vi "run_script-as_admin.vi"(8 "error in (no error)":errorcluster, 11 "script_command":string) -> (0 "error out":errorcluster)   [LabVIEW 2015, in "lv-bin-windows.lvlib" / "v1.lvlib"]
uses:
  v1.lvlib
  <userlib>/antonio-alexander/lv-bin/lv-bin/public/api/v1/v1.lvlib
  lv-bin-windows.lvlib
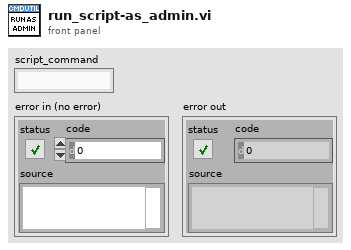
[diagram p1: front panel]
types:
  T1 = enum16{"open", "replace", "create", "open or create", "replace or create", "replace or create with confirmation"}
  T2 = typedef "lv-bin.lvlib/v1.lvlib/temp_dir_config.ctl" = cluster{"root_folder":path, "prefix":string}
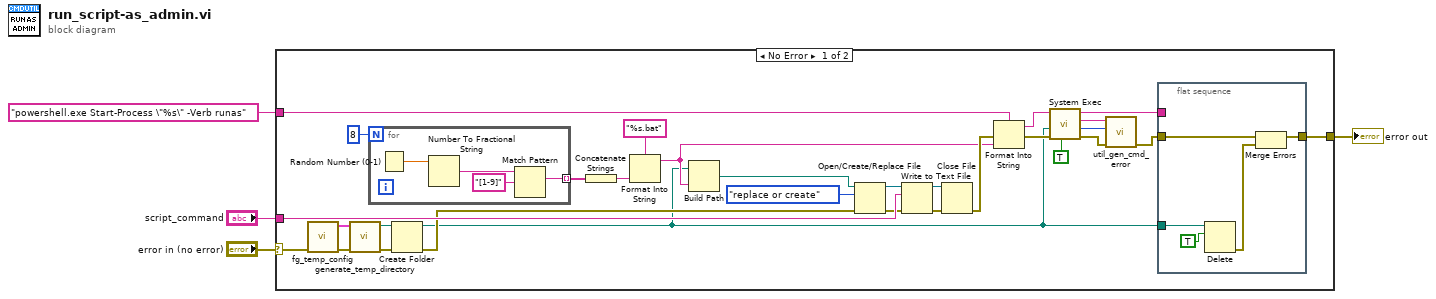
[diagram p0: block diagram]
diagram:
  n1 = case shown="No Error" "error in (no error)" {
    selector: "error in (no error)" -> [w7 w44]
    tunnel: "powershell.exe Start-Process \"%s\" -Verb runas" ("format string") -> [w34 _]
    tunnel: "script_command" -> [w25 _]
    tunnel: [w13 w44] -> w1
    frame No Error {
      n2 = call "fg_temp_config.vi"("error in (no error)"=w7) -> ("error out"=w6:errorcluster, "temp_dir_config"=w5:T2)  [unwired: 9 in]
      n3 = call <userlib>:"generate_temp_directory.vi"("error in (no error)"=w6, "configuration"=w5) -> ("error out"=w8:errorcluster, "temp_dir"=w9:path)  [unwired: 8 in]
      n4 = for {
        N: 8 -> [_]
        tunnel: [w40] -> w29 mode=indexing
        n5 = Random Number (0-1)() -> (number: 0 to 1=w43:dbl)
        n6 = Number To Fractional String(number=w43) -> (F-format string=w42:string)  [unwired: 3 in]
        n7 = Match Pattern(string=w42, regular expression="[1-9]") -> (match substring=w40:string)  [unwired: 1 in, 3 out]
      }
      n8 = Create Folder(path (use dialog)=w9, error in=w8) -> (created path=w15:path, error out=w22:errorcluster)  [unwired: 1 in, 1 out]
      n9 = Concatenate Strings(w29) -> (w27:string)
      n10 = Format Into String(format string="%s.bat", w27) -> (resulting string=w16:string)  [unwired: 2 in, 1 out]
      n11 = Build Path(base path=w15, name or relative path=w16) -> (appended path=w23:path)
      n12 = Open/Create/Replace File(file path (use dialog)=w23, error in=w22, operation (0:open)=T1."replace or create") -> (refnum out=w24:refnum<file>, error out=w21:errorcluster)  [unwired: 3 in, 1 out]
      n13 = Write to Text File(file (use dialog)=w24, text=w25, error in=w21) -> (refnum out=w20:refnum<file>, error out=w19:errorcluster)  [unwired: 1 in, 1 out]
      n14 = Close File(refnum=w20, error in=w19) -> (error out=w18:errorcluster)  [unwired: 1 out]
      n15 = Format Into String(format string=w34, error in=w18, w16) -> (resulting string=w33:string, error out=w30:errorcluster)  [unwired: 1 in]
      n16 = call <vilib>:"System Exec.vi"("run minimized? (F)"=TRUE, "error in (no error)"=w30, "working directory"=w15, "command line"=w33) -> ("error out"=w31:errorcluster, "return code"=w10:i32, "standard error"=w11:string, "standard output"=w12:string)  [unwired: 4 in]
      n17 = call <userlib>:"util_gen_cmd_error.vi"("error in (no error)"=w31, "return_code"=w10, "standard_error"=w11) -> ("error out"=w14:errorcluster)  [unwired: 8 in]
      n18 = flat-sequence {
        tunnel: w15 -> [w39]
        tunnel: w14 -> [w37]
        tunnel: [w36] -> w13
        tunnel: w12 -> [_]
        frame #0 {
          n19 = Delete(path (use dialog)=w39, entire hierarchy (F)=TRUE) -> (error out=w38:errorcluster)  [unwired: 3 in, 2 out]
          n20 = Merge Errors(w37, w38) -> (w36:errorcluster)
        }
      }
    }
    frame Error {
    }
  }
  "error out" <- w1
